vi "test Stop Listener.vi"(8 "error in (no error)":errorcluster, 11 "TestCase in":refnum<class "Test Network Stream Nested Endpoint.lvclass">) -> (0 "error out":errorcluster, 3 "TestCase out":refnum<class "Test Network Stream Nested Endpoint.lvclass">)   [LabVIEW 2020, in "Test Network Stream Nested Endpoint.lvclass"]
uses:
  Test Network Stream Nested Endpoint.lvclass
  <vilib>/addons/_JKI Toolkits/VI Tester/TestCase.llb/TestCase.lvclass
  <vilib>/ActorFramework/Stop Msg/Stop Msg.lvclass
  <vilib>/ActorFramework/Message Queue/Message Queue.lvclass
  <vilib>/ActorFramework/LastAck/Last Ack.lvclass
  <vilib>/ActorFramework/Message Dequeuer/Message Dequeuer.lvclass
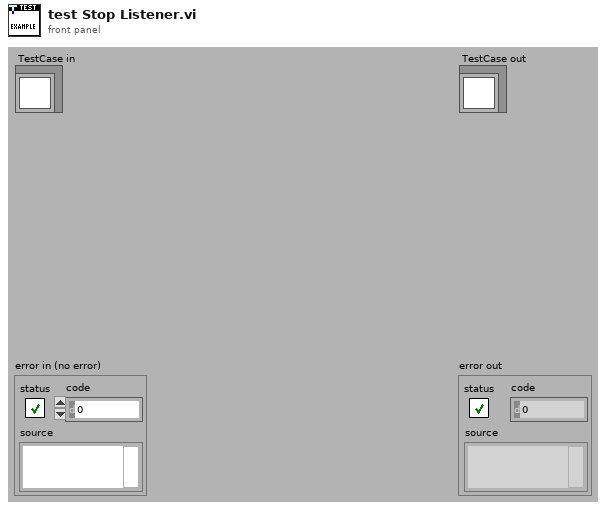
[diagram p1: front panel]
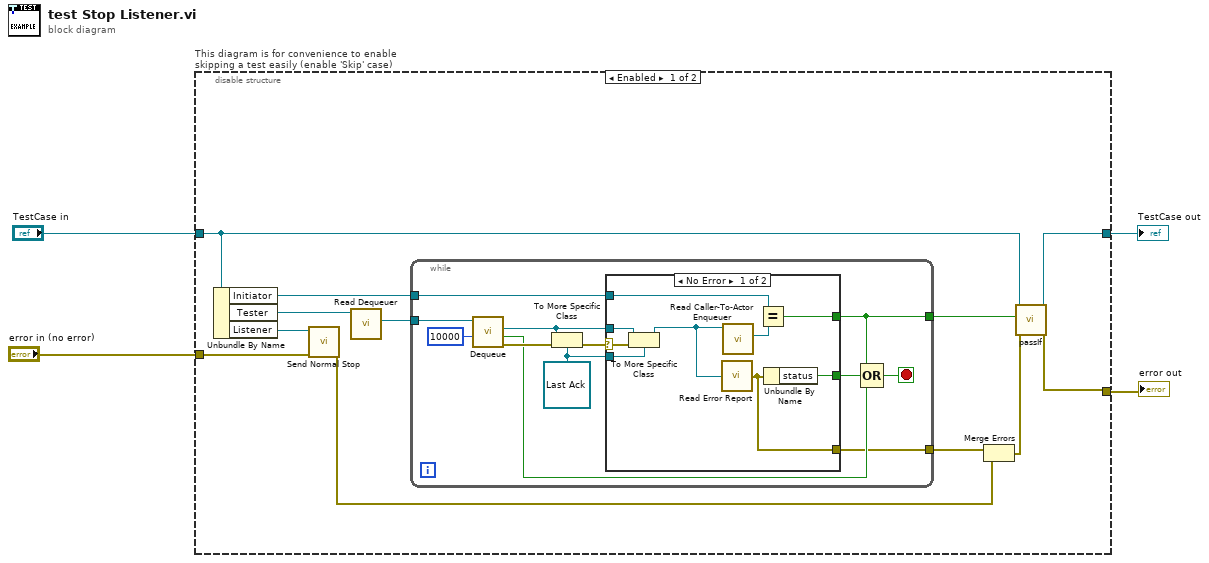
[diagram p0: block diagram]
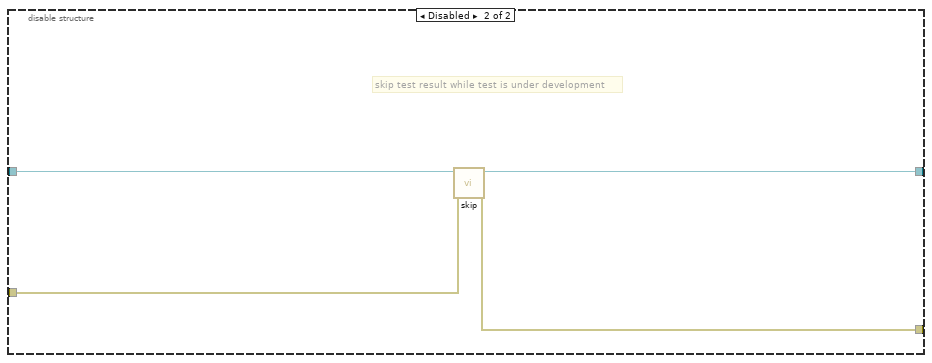
[diagram p3: hidden frame]
diagram:
  n1 = disable-structure "This diagram is for convenience to enable skipping a test easily (enable 'Skip' case)" shown="Enabled" {
    disable-tunnel: "TestCase in" -> [w14 w41]
    disable-tunnel: [w16 w39] -> w1
    disable-tunnel: [w15 w40] -> w3
    disable-tunnel: "error in (no error)" -> [w11 w38]
    frame Enabled {
      n2 = Unbundle By Name(w14) -> ("Initiator"=w8:refnum<class "Message Enqueuer.lvclass">, "Tester"=w12:refnum<class "Message Queue.lvclass">, "Listener"=w13:refnum<class "Message Enqueuer.lvclass">)
      n3 = call <vilib>:"Send Normal Stop.vi"("error in (no error)"=w11, "Message Enqueuer"=w13) -> ("error out"=w9:errorcluster)  [unwired: 9 in]
      n4 = call <vilib>:"Read Dequeuer.vi"("Message Queue"=w12) -> ("Message Dequeuer"=w7:refnum<class "Message Dequeuer.lvclass">)  [unwired: 10 in]
      n5 = while {
        tunnel: w7 -> [w28]
        tunnel: w8 -> [w25]
        tunnel: [w21] -> w6
        tunnel: [w20] -> w5
        stop <- w23 stop-if-true
        w17 = refnum<class "Last Ack.lvclass"> refnum ("Last Ack")
        n6 = call <vilib>:"Dequeue.vi"("timeout in ms (-1)"=10000, "Message Dequeuer in"=w28) -> ("error out"=w26:errorcluster, "timed out?"=w22:bool, "Message"=w18:refnum<class "Message.lvclass">)  [unwired: 5 in, 2 out]
        n7 = To More Specific Class(target class=w17, reference=w18, error in=w26) -> (error out=w19:errorcluster)  [unwired: 1 out]
        n8 = case shown="No Error" w19 {
          selector: w19 -> [w32 _]
          tunnel: w25 -> [w36 _]
          tunnel: [w35 _] -> w24
          tunnel: [w34 _] -> w21
          tunnel: [w33 _] -> w20
          tunnel: w18 -> [w31 _]
          tunnel: w17 -> [w30 _]
          frame No Error {
            n9 = To More Specific Class(target class=w30, reference=w31, error in=w32) -> (specific class reference=w29:refnum<class "Last Ack.lvclass">)  [unwired: 1 out]
            n10 = call <vilib>:"Read Error Report.vi"("Last Ack"=w29) -> ("error report"=w33:errorcluster)
            n11 = call <vilib>:"Read Caller-To-Actor Enqueuer.vi"("Last Ack"=w29) -> ("Caller-to-Actor Enqueuer"=w37:refnum<class "Message Enqueuer.lvclass">)  [unwired: 10 in]
            n12 = Equal?(x=w36, y=w37) -> (x = y?=w34:bool)
            n13 = Unbundle By Name(w33) -> ("status"=w35:bool)
          }
          frame Error {
          }
        }
        n14 = Compound Arithmetic op=OR(w21, w24, w22) -> (w23:bool)
      }
      n15 = Merge Errors(w5, w9) -> (w10:errorcluster)
      n16 = call-dynamic "passIf.vi"("error in (no error)"=w10, "pass"=w6, "TestCase in"=w14) -> ("error out"=w15:errorcluster, "TestCase out"=w16:refnum<class "Test Network Stream Nested Endpoint.lvclass">)  [unwired: 7 in]
    }
    frame Disabled {
      # "skip test result while test is under development"
      n17 = call <vilib>:"skip.vi"("error in (no error)"=w38, "TestCase in"=w41) -> ("error out"=w40:errorcluster, "TestCase out"=w39:refnum<class "Test Network Stream Nested Endpoint.lvclass">)  [unwired: 8 in]
    }
  }
  "error out" <- w3
  "TestCase out" <- w1
